vi "Mini Control Experiment.vi"(5 "Control Experiment in":refnum<class "Control Experiment.lvclass">, 6 "Username":string, 8 "error in (no error)":errorcluster, 9 "Device Description":string, 10 "Device Name":string, 11 "Base Path":path) -> (0 "error out":errorcluster, 3 "Control Experiment out":refnum<class "Control Experiment.lvclass">)   [LabVIEW 2019, in "Control Experiment.lvclass"]
uses:
  Control Experiment.lvclass
  Control Experiment.lvclass/Control Experiment.ctl
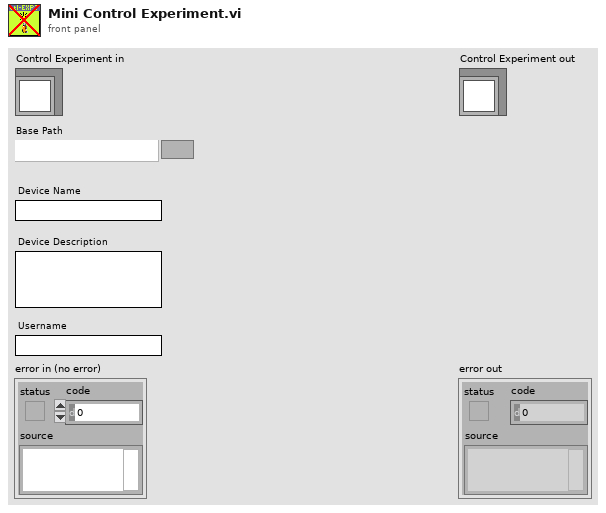
[diagram p1: front panel]
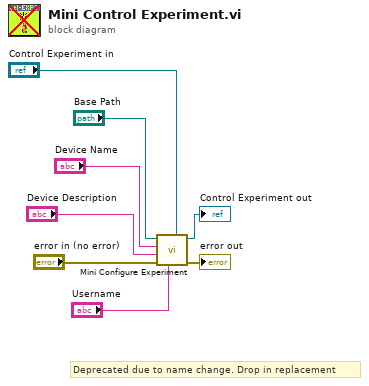
[diagram p0: block diagram]
diagram:
  # "Deprecated due to name change. Drop in replacement"
  n1 = call "Mini Configure Experiment.vi"("Control Experiment in"="Control Experiment in", "Username"="Username", "error in (no error)"="error in (no error)", "Device Description"="Device Description", "Device Name"="Device Name", "Base Path"="Base Path") -> ("error out"=→"error out":errorcluster, "Control Experiment out"=→"Control Experiment out":refnum<class "Control Experiment.lvclass">)  [unwired: 4 in]
